vi "HTTP_PostRequest.vi"() -> ()   [LabVIEW 2017]
uses:
  <vilib>/httpClient/MultipartData.ctl
  <vilib>/httpClient/LabVIEWHTTPClient.lvlib
panel:
  out "body":string
  out "headers":string
  in  "data":T1[](array[typedef])
  out "error out":errorcluster
  in  "error constant":errorcluster
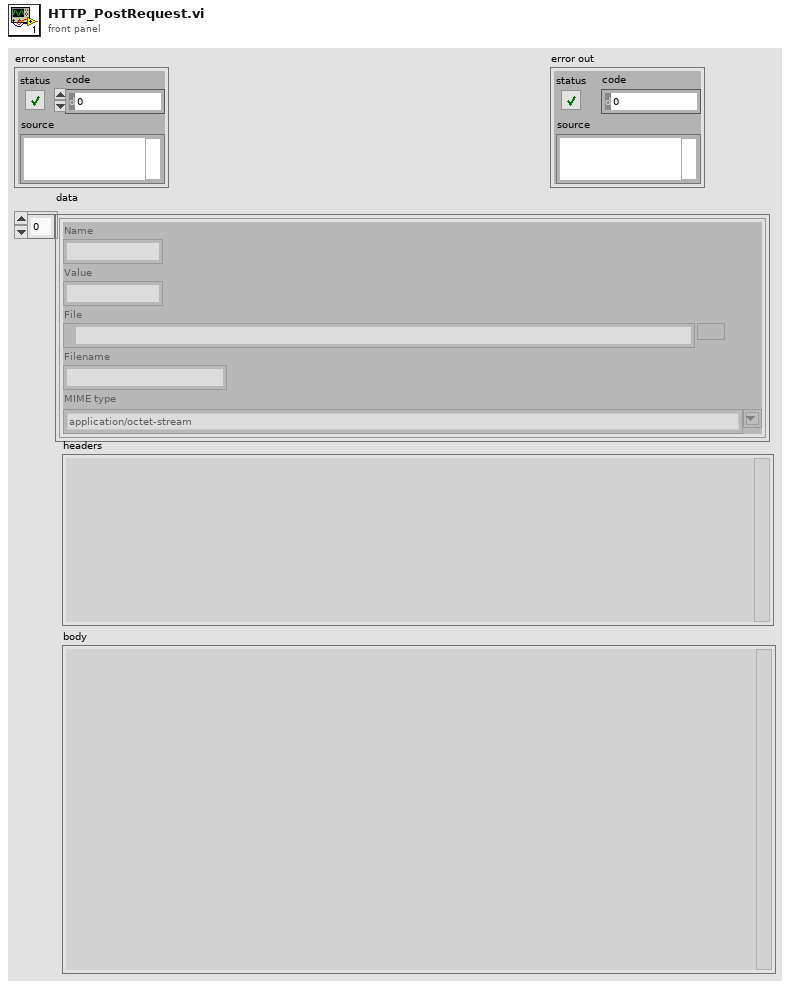
[diagram p1: front panel]
types:
  T1 = typedef "LabVIEWHTTPClient.lvlib/MultipartData.ctl" = cluster{"Name":string, "Value":string, "File":path, "Filename":string, "MIME type":string}
  T2 = typedef "LabVIEWHTTPClient.lvlib/ClientHandle.ctl" = refnum<k1>
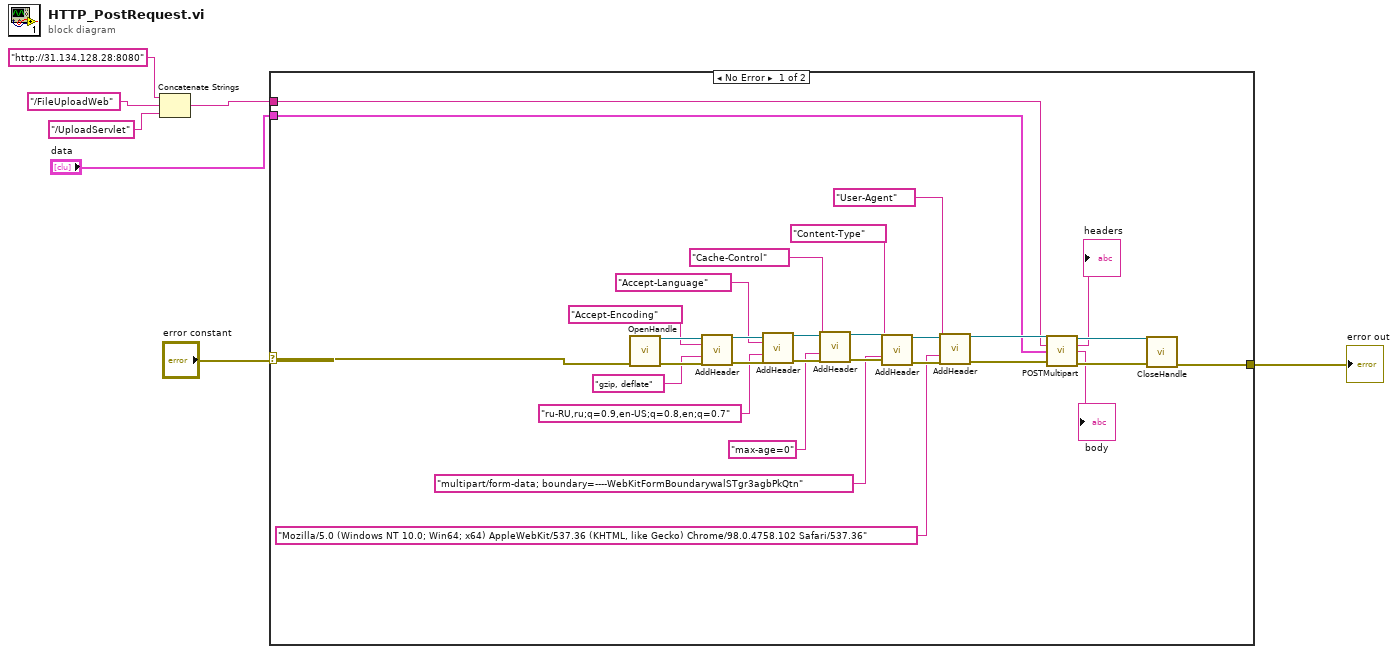
[diagram p0: block diagram]
diagram:
  n1 = Concatenate Strings("http://31.134.128.28:8080" ("url"), "/FileUploadWeb" ("url"), "/UploadServlet" ("url")) -> (w3:string)
  n2 = case shown="No Error" "error constant" {
    selector: "error constant" -> [w20 w38]
    tunnel: [w19 w38] -> w6
    tunnel: w3 -> [w18 _]
    tunnel: "data" -> [w17 _]
    frame No Error {
      n3 = call <vilib>:"OpenHandle.vi"("error in (no error)"=w20) -> ("client handle out"=w37:T2, "error out"=w32:errorcluster)  [unwired: 13 in]
      n4 = call <vilib>:"AddHeader.vi"("client handle"=w37, "header"="Accept-Encoding", "value"="gzip, deflate", "error in (no error)"=w32) -> ("client handle out"=w36:T2, "error out"=w31:errorcluster)  [unwired: 10 in]
      n5 = call <vilib>:"AddHeader.vi"("client handle"=w36, "header"="Accept-Language", "value"="ru-RU,ru;q=0.9,en-US;q=0.8,en;q=0.7", "error in (no error)"=w31) -> ("client handle out"=w35:T2, "error out"=w30:errorcluster)  [unwired: 10 in]
      n6 = call <vilib>:"AddHeader.vi"("client handle"=w35, "header"="Cache-Control", "value"="max-age=0", "error in (no error)"=w30) -> ("client handle out"=w34:T2, "error out"=w29:errorcluster)  [unwired: 10 in]
      n7 = call <vilib>:"AddHeader.vi"("client handle"=w34, "header"="Content-Type", "value"="multipart/form-data; boundary=----WebKitFormBoundarywalSTgr3agbPkQtn", "error in (no error)"=w29) -> ("client handle out"=w33:T2, "error out"=w28:errorcluster)  [unwired: 10 in]
      n8 = call <vilib>:"AddHeader.vi"("client handle"=w33, "header"="User-Agent", "value"="Mozilla/5.0 (Windows NT 10.0; Win64; x64) AppleWebKit/537.36 (KHTML, like Gecko) Chrome/98.0.4758.102 Safari/537.36", "error in (no error)"=w28) -> ("client handle out"=w27:T2, "error out"=w26:errorcluster)  [unwired: 10 in]
      n9 = call <vilib>:"POSTMultipart.vi"("client handle"=w27, "url"=w18, "data"=w17, "error in (no error)"=w26) -> ("client handle out"=w25:T2, "headers"=→"headers":string, "body"=→"body":string, "error out"=w24:errorcluster)  [unwired: 8 in]
      n10 = call <vilib>:"CloseHandle.vi"("client handle"=w25, "error in (no error)"=w24) -> ("error out"=w19:errorcluster)  [unwired: 13 in]
    }
    frame Error {
    }
  }
  "error out" <- w6
